vi "Get Sensor Scale.vi"(8 "error in (no error)":errorcluster, 10 "Sensor File Path":path, 11 "Sensor Parameter in":refnum<class "Sensor Parameter.lvclass">) -> (0 "error out":errorcluster, 1 "Intercept":dbl, 2 "Slope":dbl, 3 "Sensor Parameter out":refnum<class "Sensor Parameter.lvclass">)   [LabVIEW 2013, in "Parameter.lvlib" / "Sensor Parameter.lvclass"]
uses:
  Sensor Parameter.lvclass
  <vilib>/xml/Load XML File.vi
  <vilib>/xml/Close Reference(Node).vi
  <vilib>/xml/NI_XML.lvlib
  <vilib>/Analysis/NI_AALPro.lvlib
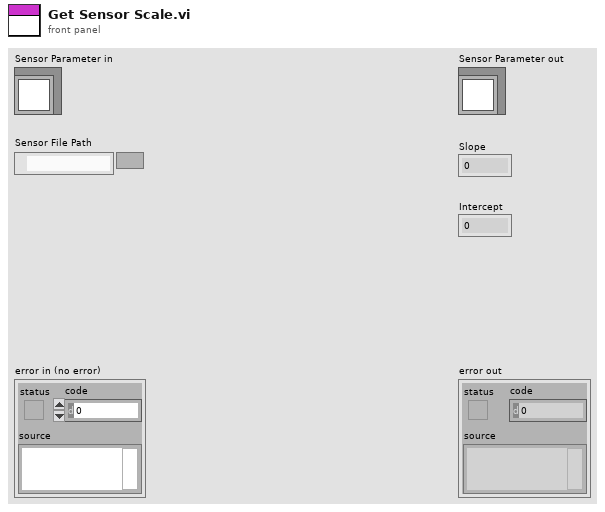
[diagram p1: front panel]
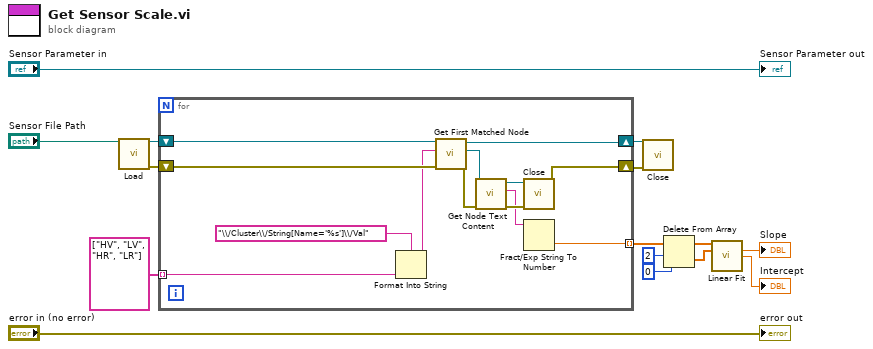
[diagram p0: block diagram]
diagram:
  n1 = call-poly <vilib>:"Load.vi"("path to XML document"="Sensor File Path") -> ("DOM document out"=w15:refnum<k20>, "error out"=w14:errorcluster)  [unwired: 12 in, 1 out]
  n2 = for {
    shift-right: [w28] -> w13
    shift-left: w15 -> [w27]
    shift-right: [w21] -> w12
    shift-left: w14 -> [w26]
    tunnel: string[] ["HV", "LV", "HR", "LR"] -> [w18] mode=indexing
    tunnel: [w16] -> w7 mode=indexing
    n3 = Format Into String(format string="\\/Cluster\\/String[Name='%s']\\/Val" ("XPath expression"), w18) -> (resulting string=w24:string)  [unwired: 2 in, 1 out]
    n4 = call <vilib>:"Get First Matched Node.vi"("error in (no error)"=w26, "XPath expression"=w24, "node in"=w27) -> ("error out"=w22:errorcluster, "node result"=w23:refnum<k20>, "node out"=w28:refnum<k20>)  [unwired: 6 in]
    n5 = call <vilib>:"Get Node Text Content.vi"("error in (no error)"=w22, "node in"=w23) -> ("error out"=w20:errorcluster, "node text"=w17:string, "node out"=w19:refnum<k20>)  [unwired: 7 in]
    n6 = call-poly <vilib>:"Close.vi"("error in (no error)"=w20, "node"=w19) -> ("error out"=w21:errorcluster)  [unwired: 7 in]
    n7 = Fract/Exp String To Number(string=w17) -> (number=w16:dbl)  [unwired: 3 in, 1 out]
  }
  n8 = call-poly <vilib>:"Close.vi"("error in (no error)"=w12, "node"=w13) -> ()  [unwired: 7 in, 1 out]
  n9 = Delete From Array(array=w7, length=2, index=0) -> (deleted portion=w3:dbl[], array with subset deleted=w4:dbl[])
  n10 = call <vilib>:"Linear Fit.vi"("Y"=w4, "X"=w3) -> ("slope"=→"Slope":dbl, "intercept"=→"Intercept":dbl)  [unwired: 9 in, 3 out]
  "error out" <- "error in (no error)"
  "Sensor Parameter out" <- "Sensor Parameter in"
